vi "Diff_Drive_System_Set_Auto.vi"(11 "Auto Mode":bool) -> ()   [LabVIEW 2019]
uses:
  Diff_Drive_System_Globals.vi
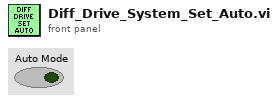
[diagram p1: front panel]
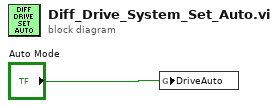
[diagram p0: block diagram]
diagram:
  n1 = global write "Diff_Drive_System_Globals.vi" "DriveAuto"("Auto Mode") -> ()
